vi "TempCtl.vi"(2 "shiftReg":bool, 3 "enable":bool, 4 "Hysterese":sgl, 5 "Soll":sgl, 6 "IST":dbl, 7 "heating":bool) -> (0 "shiftReg":bool, 1 "heating":bool)   [LabVIEW 2011]
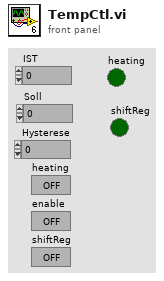
[diagram p1: front panel]
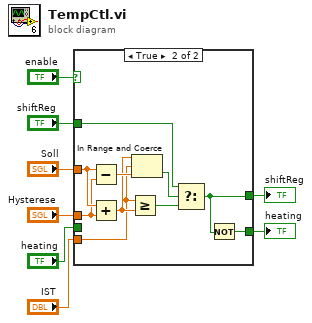
[diagram p0: block diagram]
diagram:
  n1 = case shown="True" "enable" {
    tunnel: "Soll" -> [_ w16]
    tunnel: "Hysterese" -> [_ w15]
    tunnel: [w10 w14] -> w1
    tunnel: "heating" -> [w10 _]
    tunnel: "IST" -> [_ w13]
    tunnel: "shiftReg" -> [w9 w12]
    tunnel: [w9 w11] -> w7
    frame False {
    }
    frame True {
      n2 = Subtract(x=w16, y=w15) -> (x-y=w20:sgl)
      n3 = Add(x=w16, y=w15) -> (x+y=w18:sgl)
      n4 = Greater Or Equal?(x=w13, y=w18) -> (x >= y?=w17:bool)
      n5 = In Range and Coerce(upper limit=w18, x=w13, lower limit=w20) -> (In Range?=w19:bool)  [unwired: 1 out]
      n6 = Select(t=w12, s=w19, f=w17) -> (s? t:f=w11:bool)
      n7 = Not(x=w11) -> (.not. x?=w14:bool)
    }
  }
  "shiftReg" <- w7
  "heating" <- w1
